vi "handle tracker.vi"() -> ()   [LabVIEW 2020]
uses:
  client/client.lvlib
panel:
  out "error out":errorcluster
  in  "Stop":bool
  out "buf out":string
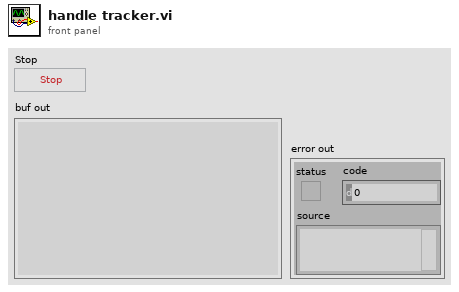
[diagram p1: front panel]
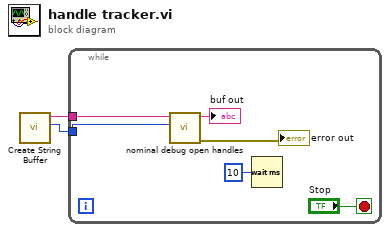
[diagram p0: block diagram]
diagram:
  n1 = call "Create String Buffer.vi"() -> ("dub Buffer Size"=w1:i32, "String Buffer"=w2:string)  [unwired: 9 in, 1 out]
  n2 = while {
    tunnel: w2 -> [w8]
    tunnel: w1 -> [w7]
    stop <- "Stop" stop-if-true
    n3 = call "nominal debug open handles.vi"("cap"=w7, "buf"=w8) -> ("error out"=→"error out":errorcluster, "buf out"=→"buf out":string)  [unwired: 6 in, 2 out]
    n4 = Wait (ms)(milliseconds to wait=u32 10) -> ()  [unwired: 1 out]
  }
